vi "Project Data Initial for manual.vi"(10 "VISA resource name":refnum<visa-resource-name>="COM1", 11 "configuration file path":path=path "C:/Users/MyUser/Desktop/S2_Project.txt") -> (0 "error out":errorcluster, 1 "Step Content":string[][](table), 2 "Retry":i32, 3 "process cluster":cluster{string[], i32[]})   [LabVIEW 2019]
uses:
  <vilib>/Utility/config.llb/Read Key (String).vi
  Global/Process Global.vi
  <vilib>/Utility/config.llb/NI_LVConfig.lvlib
  Ctrl/StationCmdSelect.ctl
  FlowCtrl Class/LineScan/LineScan.lvclass
  Ctrl/MeasureDisplayTab.ctl
  LLB/Commonly VI/Main Glb.vi
  LLB/Commonly VI.lvlib
  Ctrl/Table Save.ctl
  Ctrl/Auto Inspection Station Name2.ctl
  Ctrl/Auto Inspection Data Name.ctl
  Ctrl/S2 Station IO.ctl
panel:
  out "ToolStringOut_P1_2":string
  out "P1 Receive":string[](array[string])
  out "ToolStringOut_P1":string
  out "Initial_ChkSum":string
  out "Array":string[](array[string])
  out "S1 ChkSum":string
  out "ToolStringOut_Init":string
  out "S1 ToolStringOut":string
  out "Initial receive 2":string
  out "result string 2":string
  out "Program receive 2":string
  out "S2 receive":string
  out "Blue Scan2 receive":string
  out "T2 buffer":string
  out "T2 μA":dbl format="%#_6f"
  out "T1 buffer":string
  out "T1 μA":dbl format="%#_6f"
  in  "error in (no error)":errorcluster
  out "Blue Scan receive":string
  out "S1 receive":string
  out "Program receive":string
  out "Initial receive":string
  out "Act Step":i32
  out "retry次數":string[](array[string])
  in  "stop":bool
  out "Boolean":bool=TRUE
  in  "Numeric 3":i32
  out "format receive":string
  out "CurrentCmd":string
  out "Numeric":dbl
  in  "Table Control":string[][](table)=[["PCBA BARCODE", ""], ["硬體(Tool初始化)", ""], ["company(Tool初始化)", ""], ["耗電流 uA(電流表)", "T"], ["電池負載電壓", "T"], ["晶片ID(Tool FORMAT)", "F"], ["雷雕ID(TOOl scan、藍芽接收器)", "S"], ["Format(Tool FORMAT)", "F"], ["Programe(Tool Programe)", "P"]]
  out "subarray":string[](array[string])
  out "array":string[](array[string])
  out "Process":string[](array[string])
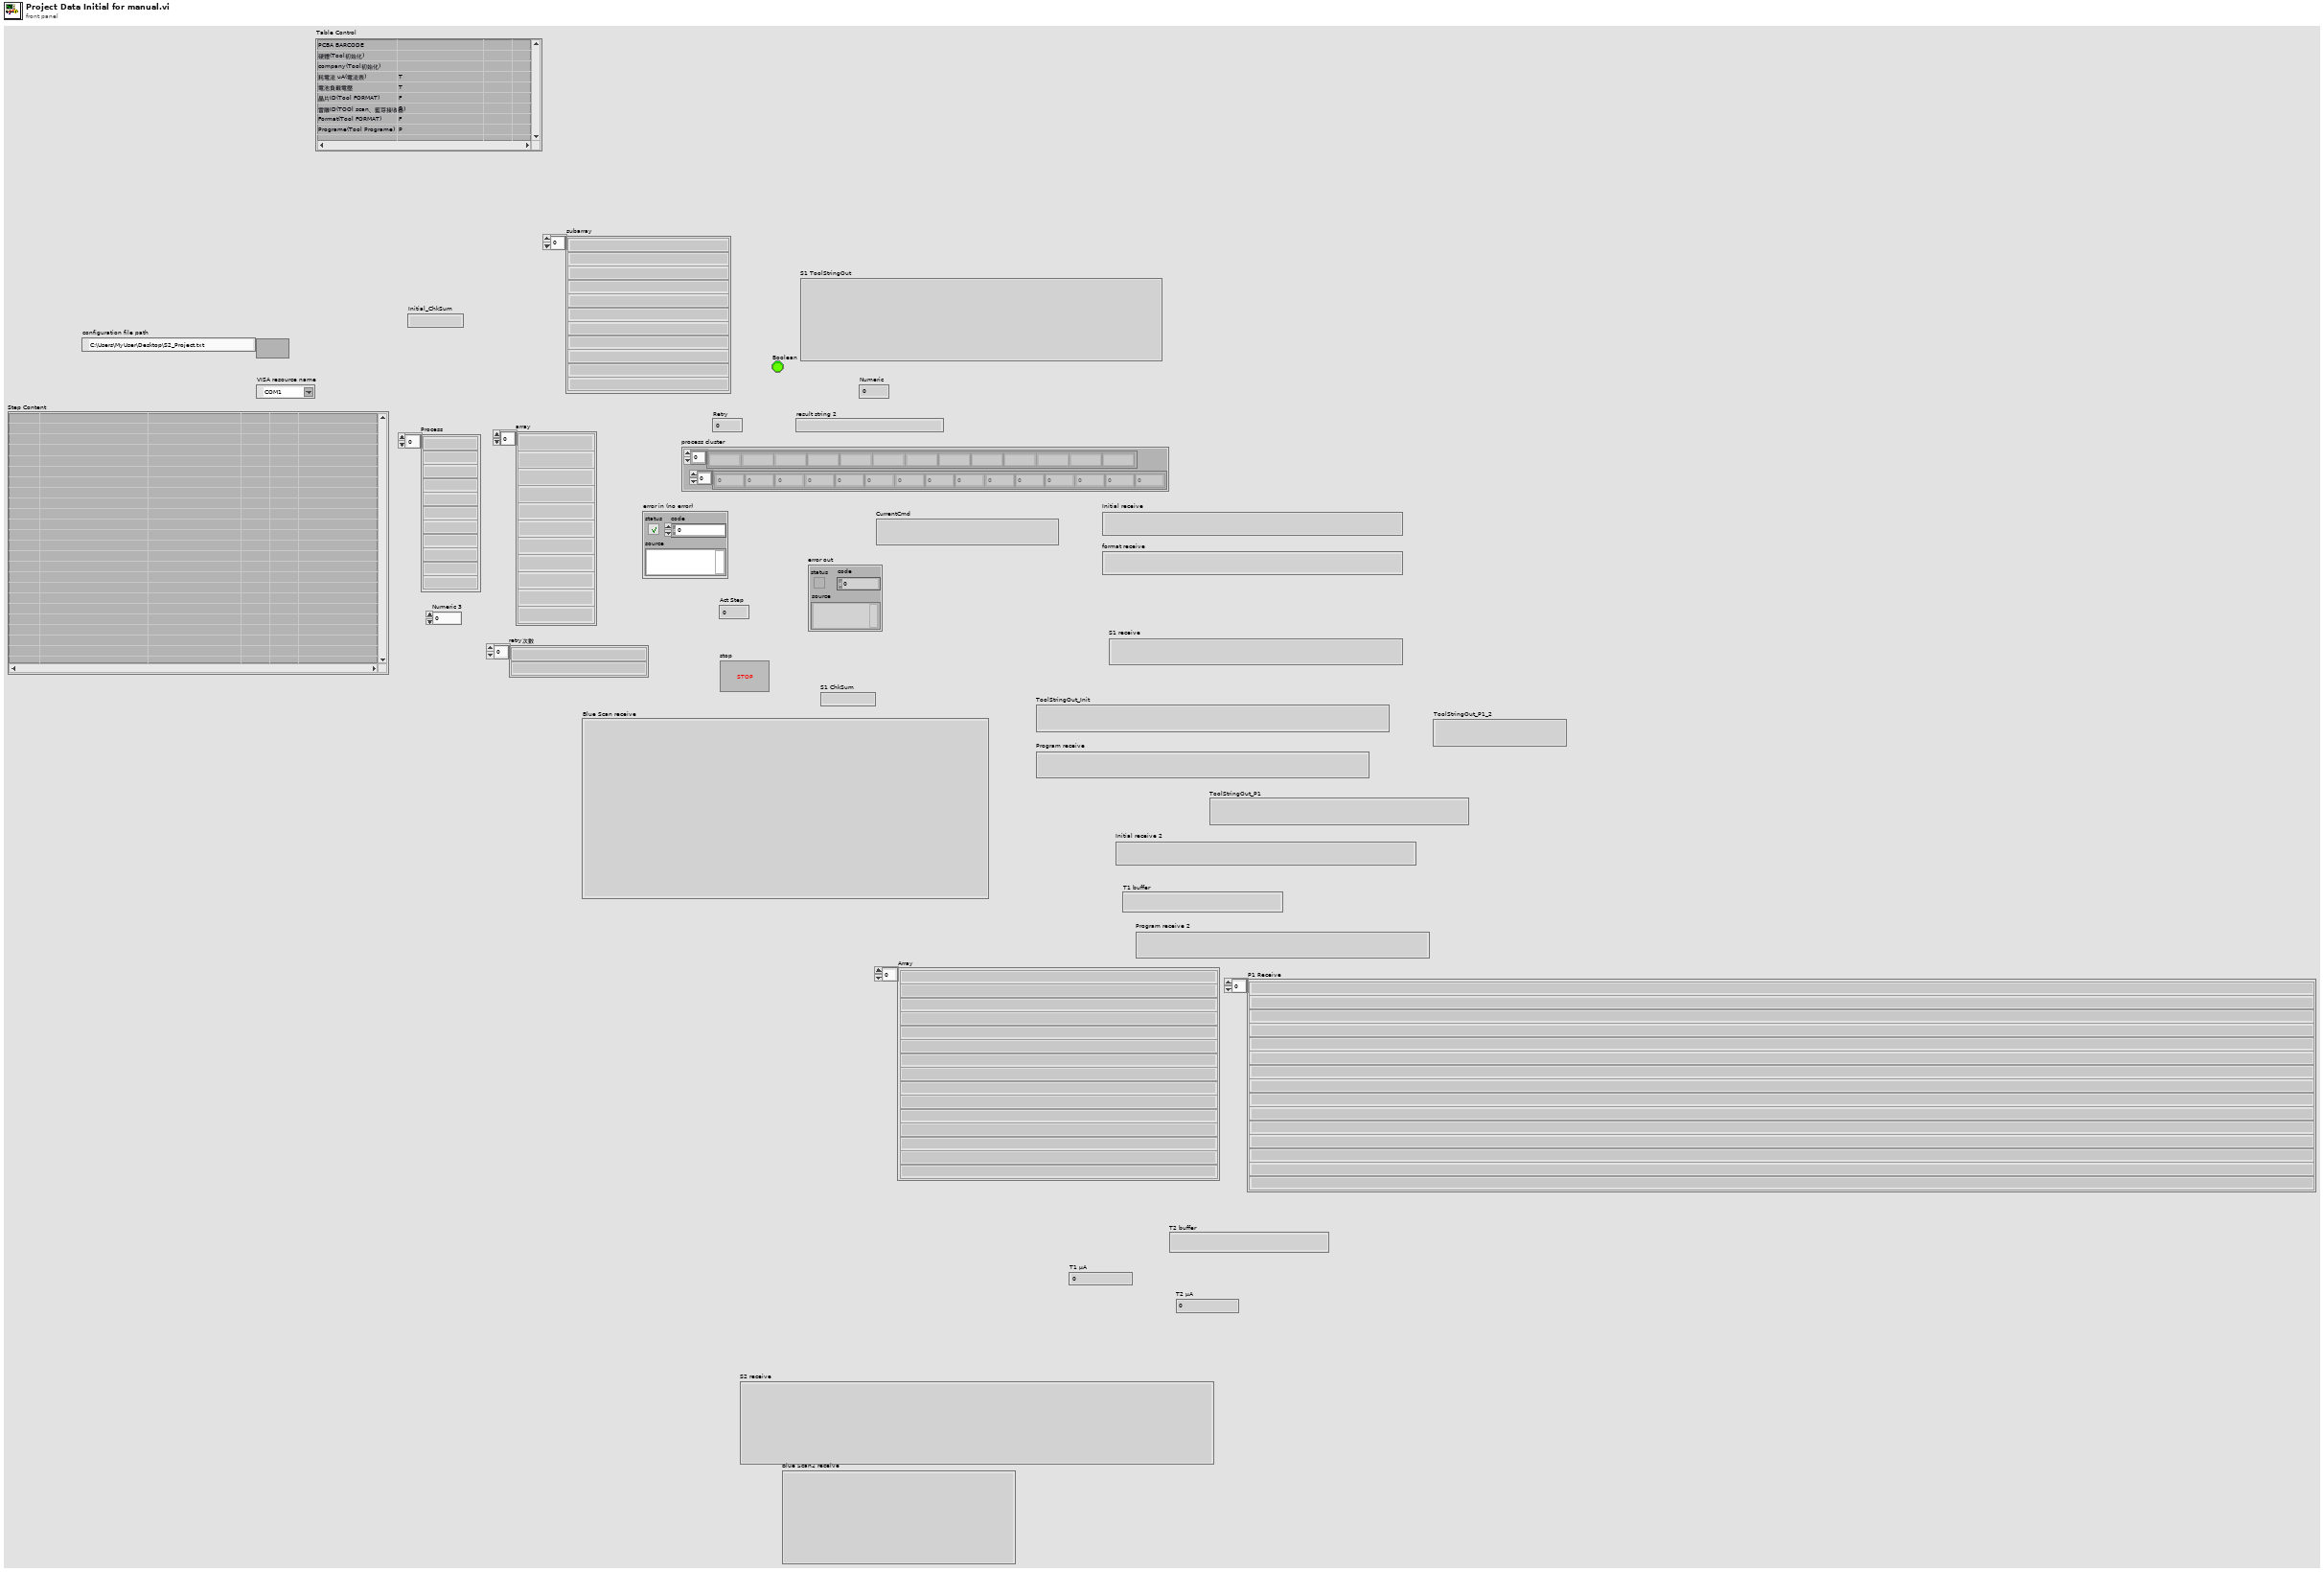
[diagram p1: front panel]
types:
  T1 = typedef "NI_LVConfig.lvlib/Config Data RefNum.ctl" = refnum<k1>
  T2 = typedef "StationCmdSelect.ctl" = enum16{"Action", "Command", "Return", "DTime", "Retry"}
  T3 = typedef "Auto Inspection Data Name.ctl" = enum16{"LocalRun", "ItemSN(TimeCode)", "CurrentAction", "Error", "Data", "OKNG", "電壓值", "電壓值判斷", "電流值", "電流值判斷", "Laser1 Data", "Laser2 Data", "Laser OKNG", "StationNO"}
  T4 = typedef "Auto Inspection Station Name2.ctl" = enum16{"S1Barcode", "S2Measure", "S3Measure", "S4Measure", "S5Measure", "S11_LaserCheck"}
  T5 = typedef "Table Save.ctl" = enum16{"initial", "Add", "Write", "Replace", "Delete", "REad", "RedTable", "Load"}
  T6 = typedef "MeasureDisplayTab.ctl" = enum16{"Tray Barcode", "PCBA BARCODE", "硬體(Tool初始化)", "company(Tool初始化)", "耗電流 uA(電流表)", "電池負載電壓", "晶片ID(Tool FORMAT)", "雷雕ID(TOOl scan、藍芽接收器)", "Format(Tool FORMAT)", "Programe(Tool Programe)", "MAC(藍芽接收器)", "ID(藍芽接收器)", "KPA(藍芽接收器)", "溫度(藍芽接收器)", "SENSOR電池電壓(藍芽接收器)", "RSSI(藍芽接收器)", "SensorType_315(FSK scan)", "FSKsnVol_315(FSK scan)", "FSKscanl_315(FSK scan)", "P_315(FSK scan)", "T_315(FSK scan)", "SensorType_433(ASK scan)", "ASKsnVol_433(ASK scan)", "ASKscan_433(ASK scan)", "P_433(ASK scan)", "T_433(ASK scan)", "測高Data"}
  T7 = typedef "S2 Station IO.ctl" = enum16{"S2站PC動作中_20", "電流量測完成產品OK_21", "電流量測完成產品NG_22", "S2站Format 執行_23", "S2 Format OK_24", "S2 Format NG_25", "S2站燒入執行_26", "S2站燒入OK_27", "S2站燒入NG_28", "S2站動作完成_29", "S3 PC動作中_30", "S3 Format 此站執行_31", "S3 Format OK_32", "S3 Format NG_33", "S3 燒入程式 此站執行_34", "S3 燒入程式 OK_35", "S3 燒入程式 NG_36", "S3 備用_37", "S3 備用_38", "S3 動作完成_39", "S4 PC動作中_40", "S4 量測完成 產品正常_41", "S4 量測完成 產品NG_42", "S4 Format 此站執行_43", "S4 Format OK_44", "S4 Format NG_45", "S4 燒入 此站不執行_46", "S4 燒入程式 OK_47", "S4 燒入程式 NG_48", "S4 藍芽Scan OK_49", "S4 藍芽Scan NG_50", "S4 動作完成_51", "給PLC要量電流訊號", "給PLC要量電壓訊號"}
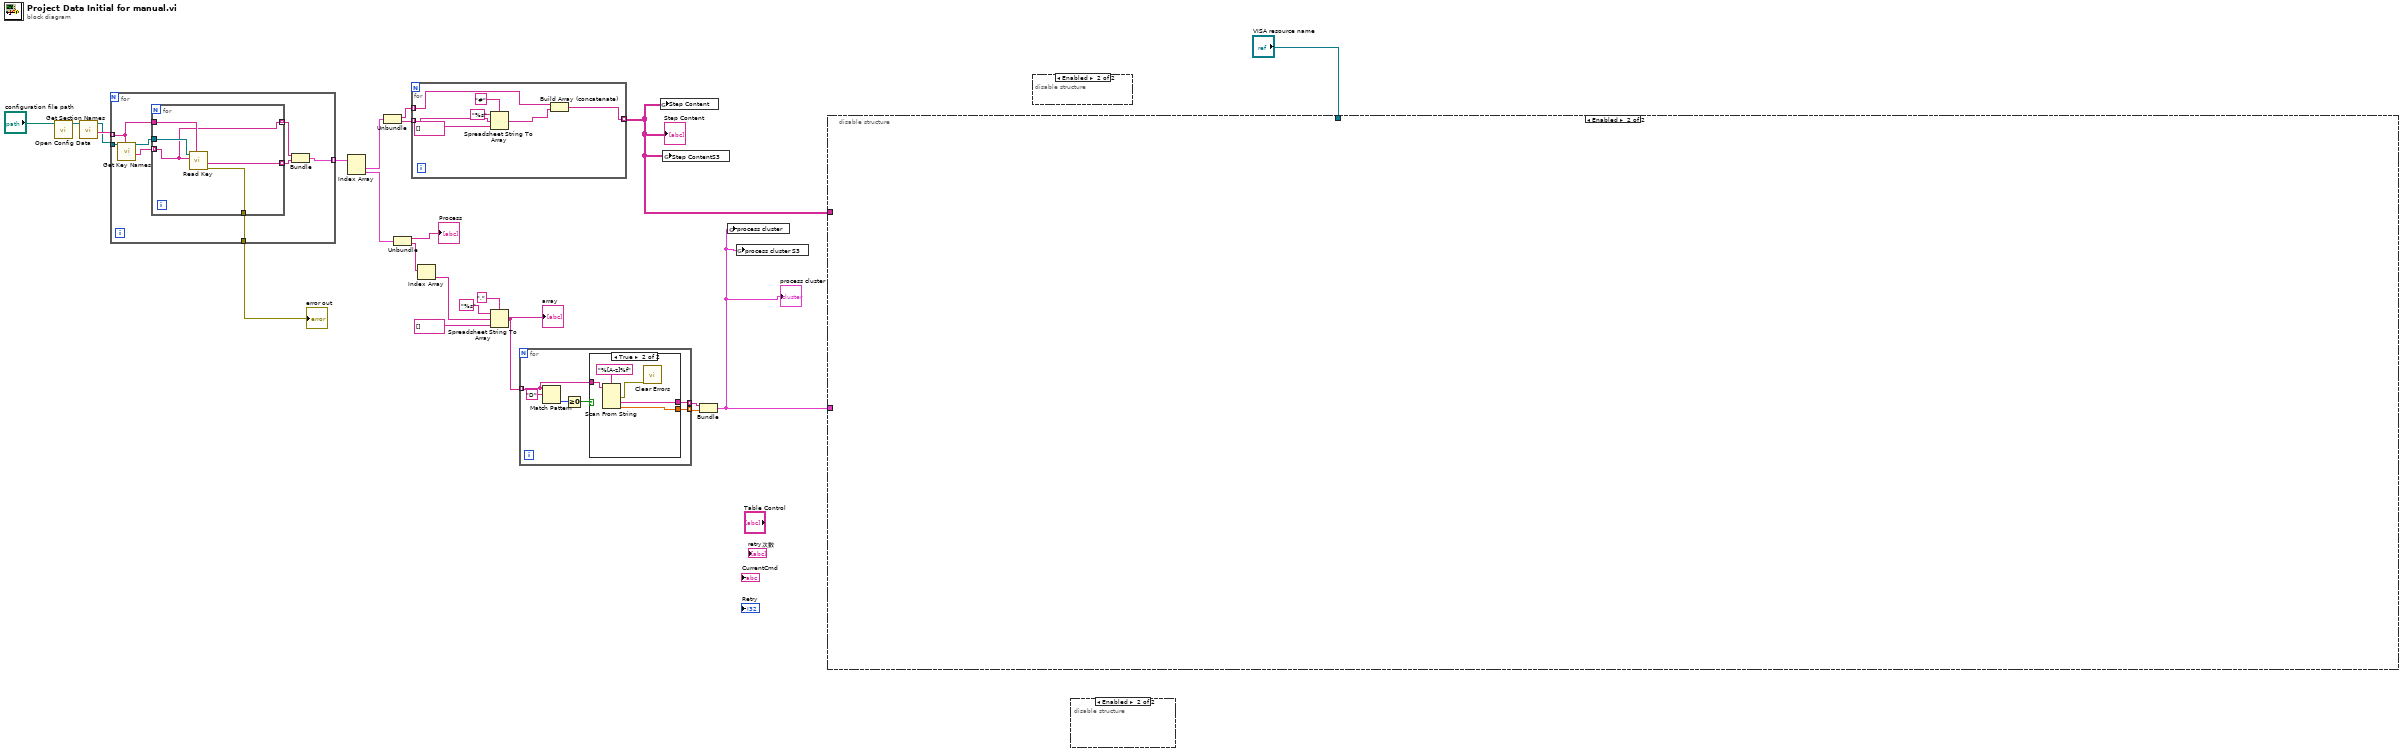
[diagram p0: block diagram]
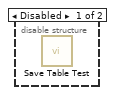
[diagram p2: hidden frame]
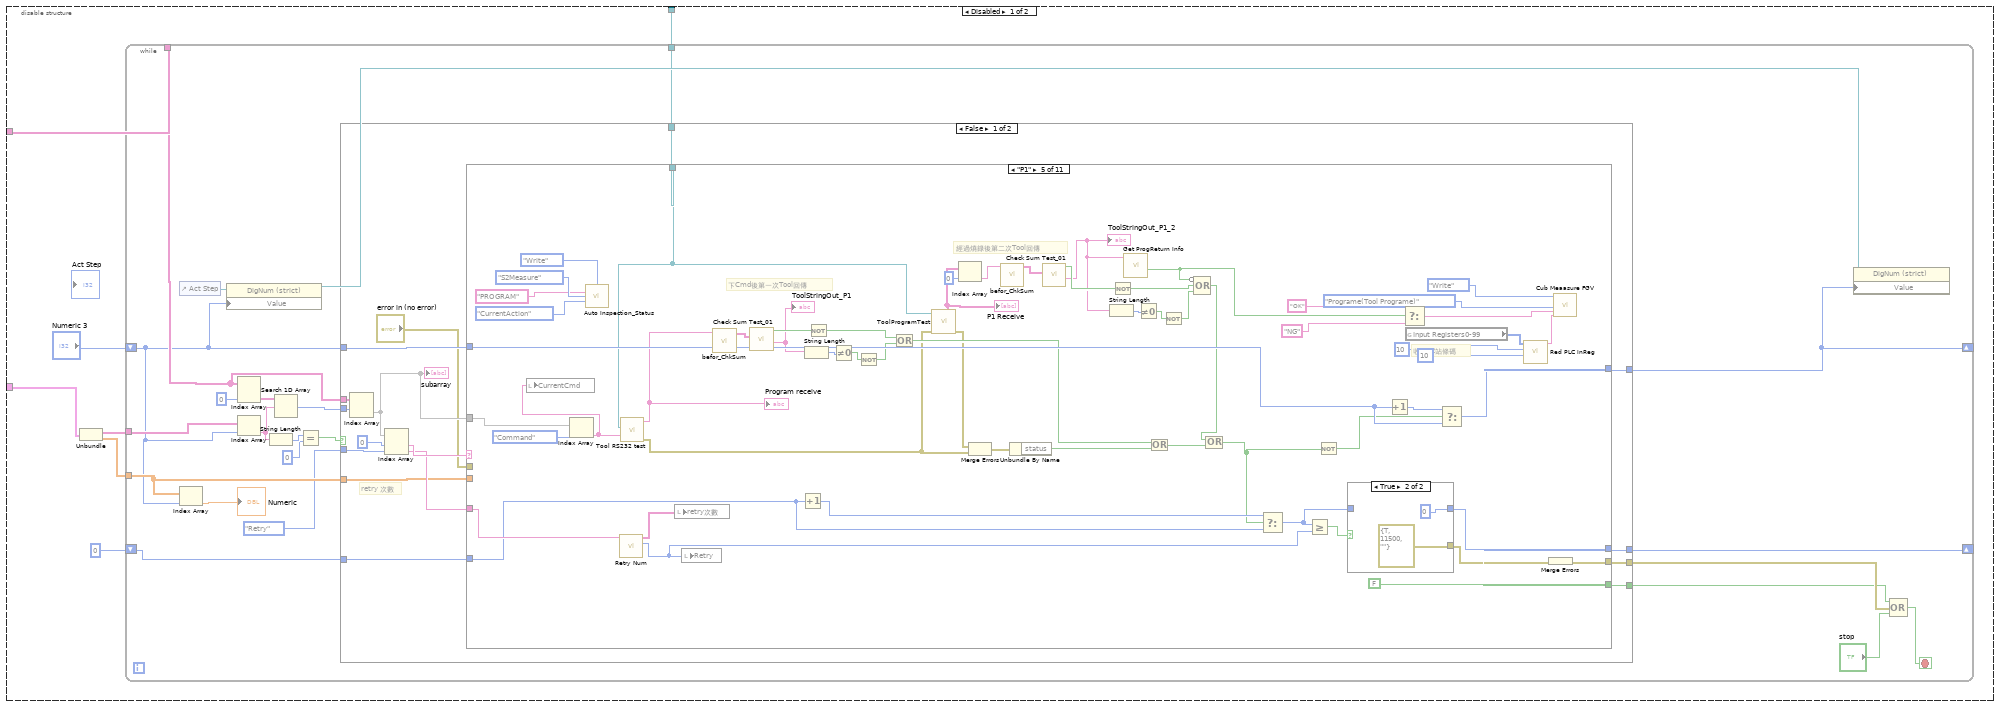
[diagram p3: hidden frame]
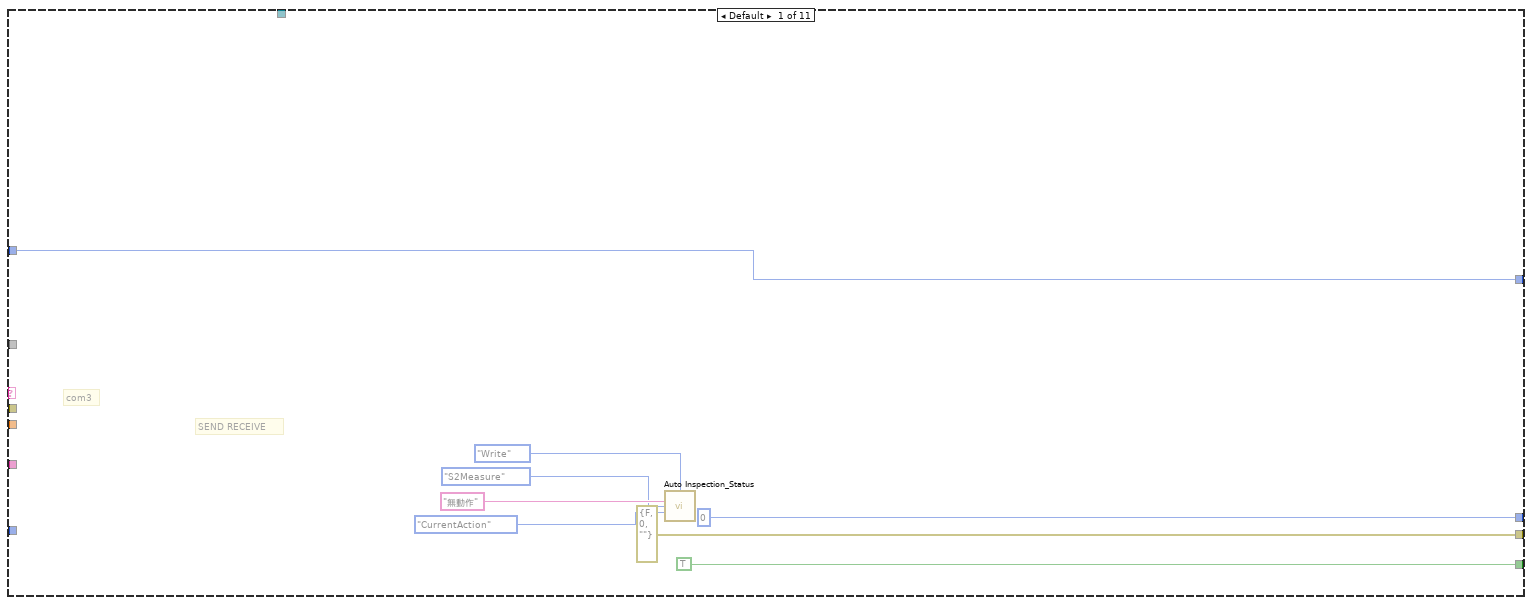
[diagram p4: hidden frame]
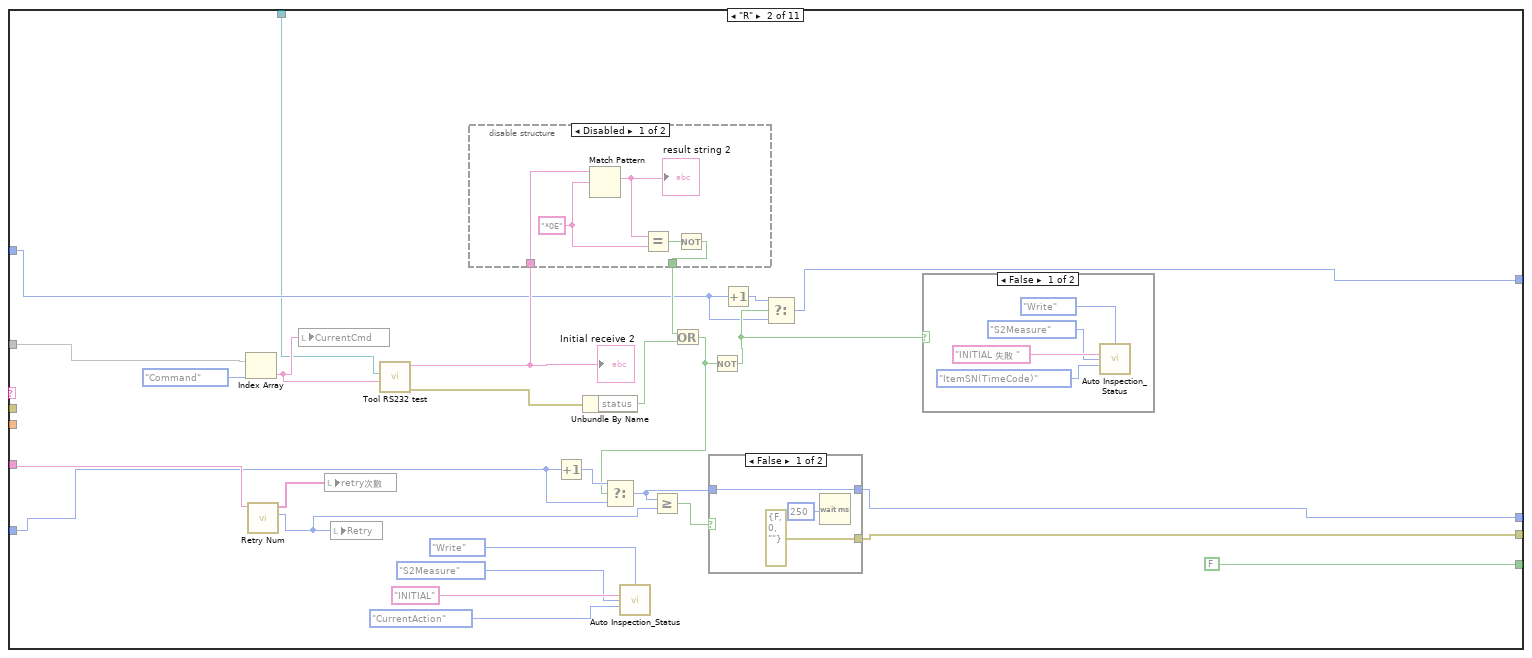
[diagram p5: hidden frame]
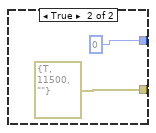
[diagram p8: hidden frame]
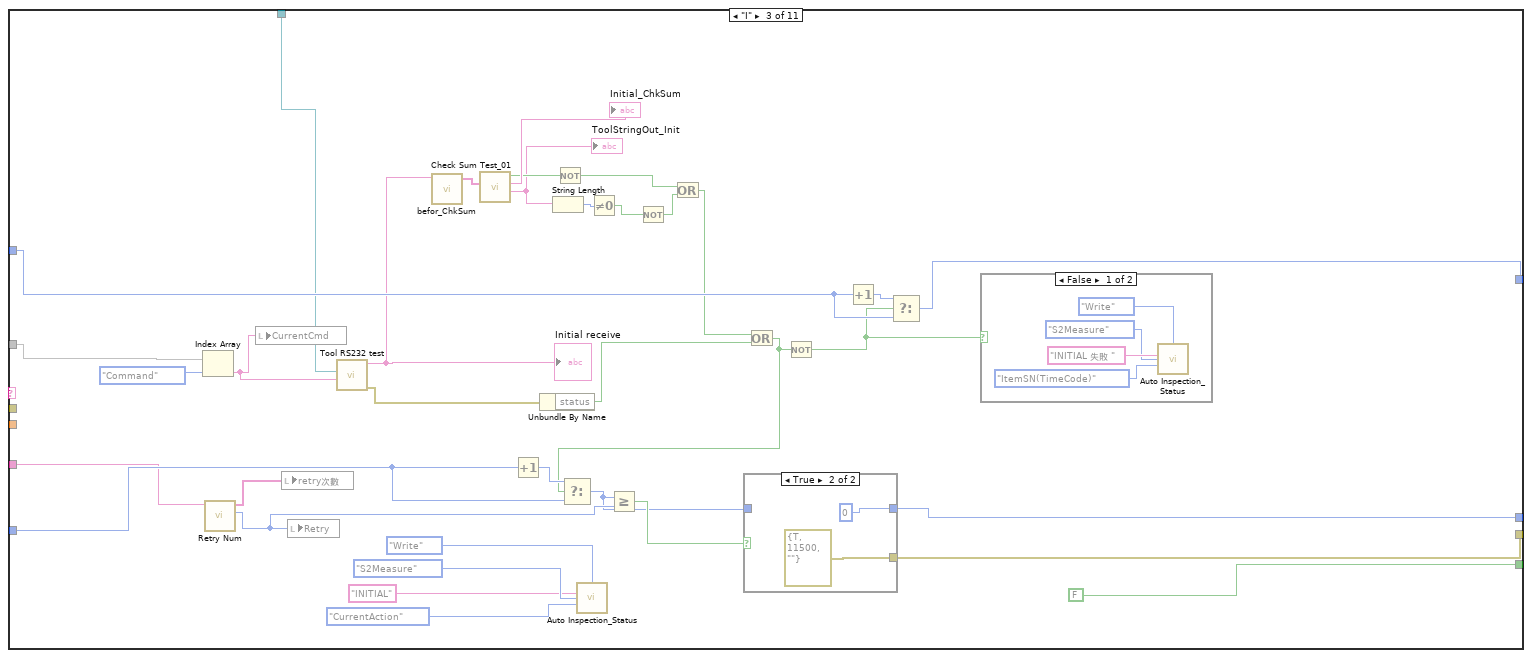
[diagram p9: hidden frame]
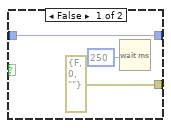
[diagram p11: hidden frame]
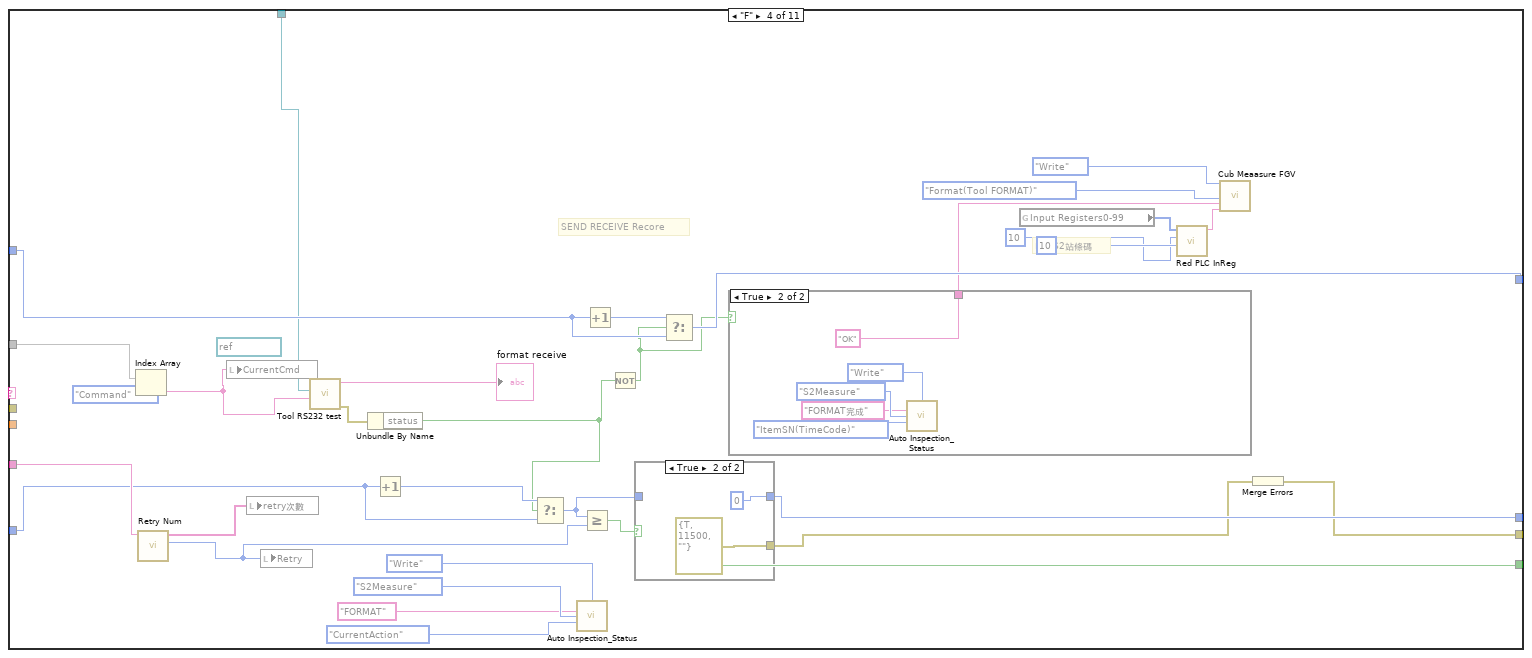
[diagram p12: hidden frame]
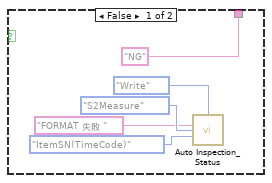
[diagram p13: hidden frame]
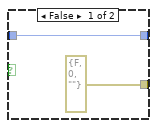
[diagram p14: hidden frame]
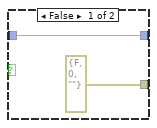
[diagram p15: hidden frame]
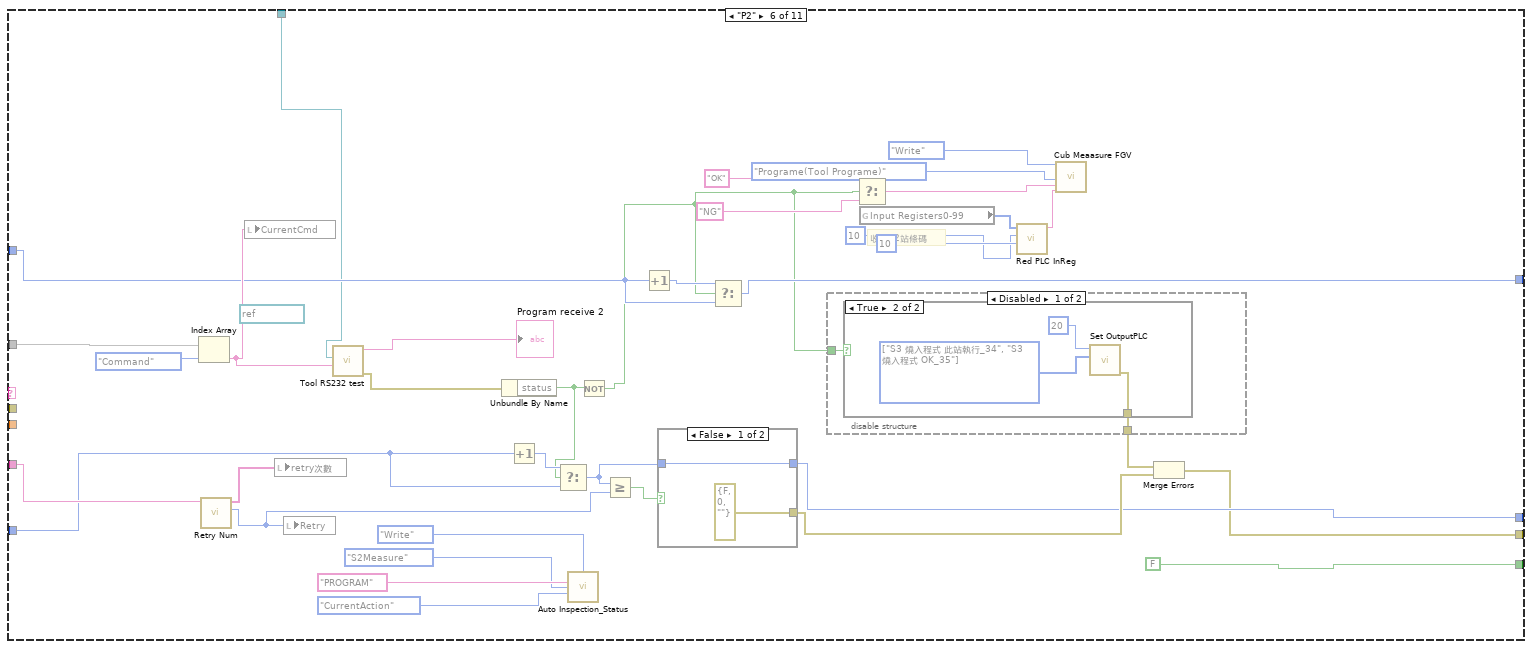
[diagram p16: hidden frame]
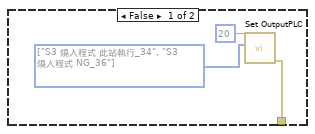
[diagram p17: hidden frame]
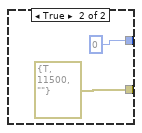
[diagram p19: hidden frame]
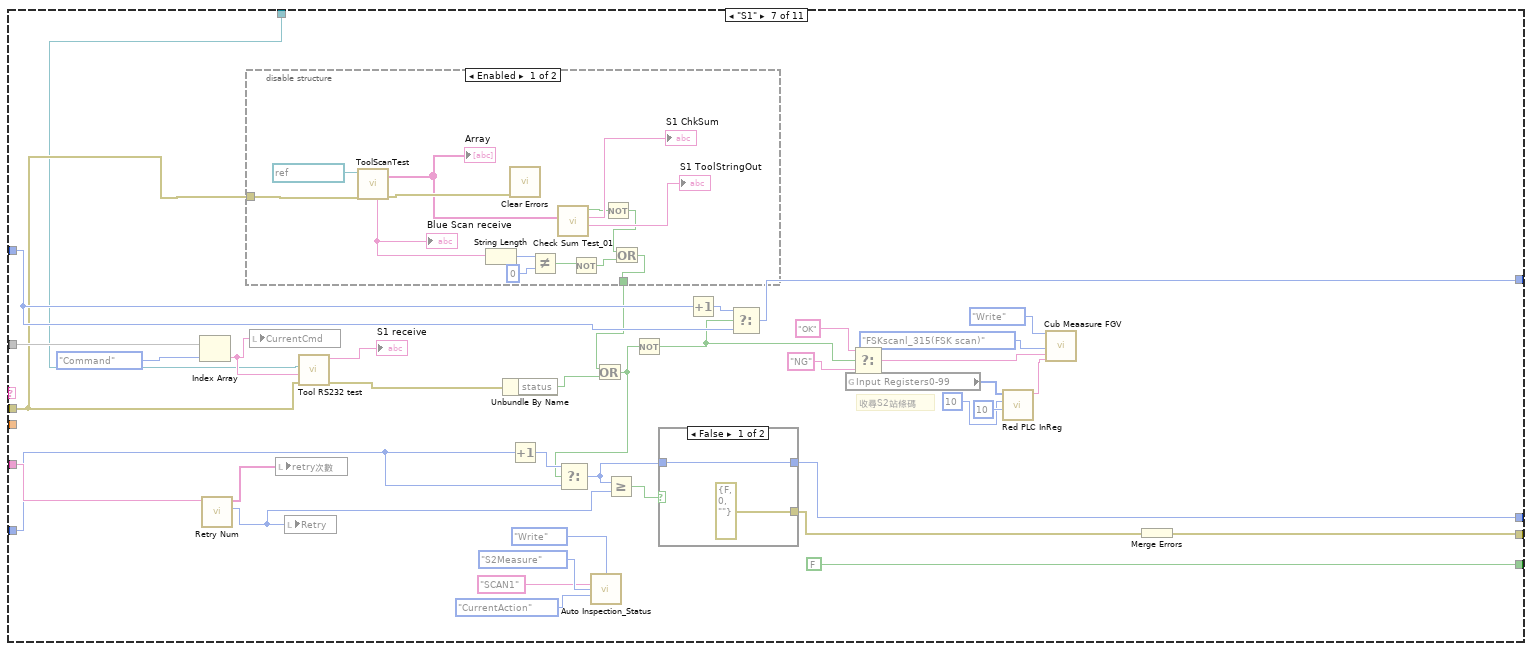
[diagram p20: hidden frame]
diagram:
  n1 = call <vilib>:"Open Config Data.vi"("configuration file path"="configuration file path") -> ("refnum"=w21:T1)  [unwired: 8 in, 2 out]
  n2 = call <vilib>:"Get Section Names.vi"("refnum"=w21) -> ("section names"=w20:string[], "refnum out"=w19:T1)  [unwired: 8 in, 1 out]
  n3 = for {
    tunnel: w19 -> [w30]
    tunnel: w20 -> [w25] mode=indexing
    tunnel: [w27] -> w17 mode=indexing
    tunnel: [w23] -> w3
    n4 = call <vilib>:"Get Key Names.vi"("section"=w25, "refnum"=w30) -> ("key names"=w29:string[], "refnum out"=w26:T1)  [unwired: 6 in, 2 out]
    n5 = for {
      tunnel: w29 -> [w32] mode=indexing
      tunnel: [w35] -> w28 mode=indexing
      tunnel: w26 -> [w34]
      tunnel: w25 -> [w33]
      tunnel: [w32] -> w24 mode=indexing
      tunnel: [w31] -> w23
      n6 = call-poly <vilib>:"Read Key.vi"("section"=w33, "key"=w32, "refnum"=w34) -> ("error out"=w31:errorcluster, "value"=w35:string)  [unwired: 5 in, 2 out]
    }
    n7 = Bundle(w24, w28) -> (w27:cluster{string[], string[]})  [unwired: 1 in]
  }
  "error out" <- w3
  n8 = Index Array(array=w17) -> (element #1=w13:cluster{string[], string[]}, element #2=w16:cluster{string[], string[]})  [unwired: 2 in]
  n9 = Unbundle(w13) -> (w14:string[], w15:string[])
  n10 = Unbundle(w16) -> (→"Process":string[], w9:string[])
  n11 = for {
    tunnel: w15 -> [w40] mode=indexing
    tunnel: [w36] -> w4 mode=indexing
    tunnel: w14 -> [w37] mode=indexing
    n12 = Spreadsheet String To Array(delimiter (Tab)="#", format string="%s", spreadsheet string=w40, array type (2D Dbl)=string[] []) -> (array=w38:string[])
    n13 = Build Array (concatenate)(w37, w38) -> (w36:string[])
  }
  "Step Content" <- w4
  n14 = Index Array(array=w9) -> (element=w8:string)  [unwired: 1 in]
  n15 = Spreadsheet String To Array(delimiter (Tab)=",", format string="%s", spreadsheet string=w8, array type (2D Dbl)=string[] []) -> (array=w7:string[])
  "array" <- w7
  n16 = for {
    tunnel: w7 -> [w43] mode=indexing
    tunnel: [w48] -> w6 mode=indexing
    tunnel: [w47] -> w5 mode=indexing
    n17 = Match Pattern(string=w43, regular expression="D") -> (offset past match=w45:i32)  [unwired: 1 in, 3 out]
    n18 = Greater Or Equal To 0?(x=w45) -> (x >= 0?=w44:bool)
    n19 = case shown="True" w44 {
      tunnel: [w50 w54] -> w48
      tunnel: [-1.0 w53] -> w47
      tunnel: w43 -> [w50 w51]
      frame False {
      }
      frame True {
        n20 = Scan From String(format string="%[A-z]%f", input string=w51) -> (error out=w52:errorcluster, output 1=w54:string, output 2=w53:dbl)  [unwired: 4 in, 2 out]
        n21 = call <vilib>:"Clear Errors.vi"("error in (no error)"=w52) -> ()  [unwired: 5 in, 2 out]
      }
    }
  }
  n22 = global write "Process Global.vi" "Step Content"(w4) -> ()
  n23 = global write "Process Global.vi" "Step ContentS3"(w4) -> ()
  n24 = Bundle(w6, w5) -> (w1:cluster{string[], dbl[]})  [unwired: 1 in]
  "process cluster" <- w1
  n25 = global write "Process Global.vi" "process cluster"(w1) -> ()
  n26 = global write "Process Global.vi" "process cluster S3"(w1) -> ()
  n27 = disable-structure shown="Enabled" {
    disable-tunnel: w4 -> [w60 _]
    disable-tunnel: w1 -> [w59 _]
    disable-tunnel: "VISA resource name" -> [w56 _]
    frame Disabled {
      n28 = Unbundle(w59) -> (w62:string[], w61:dbl[])
      n29 = while {
        tunnel: w62 -> [w85]
        tunnel: w61 -> [w84]
        tunnel: w60 -> [w83]
        shift-right: [w66] -> _
        shift-left: 0 -> [w70]
        shift-right: [w67] -> _
        shift-left: "Numeric 3" -> [w64]
        tunnel: w56 -> [w63]
        stop <- w71 stop-if-true
        n30 = control-ref of="Act Step"() -> (w69:refnum<vi>)
        n31 = Index Array(array=w84, index=w64) -> (element=→"Numeric":dbl)
        n32 = property class="DigNum (strict)"(reference=w69, "Value"=w64) -> (reference out=w68:refnum<vi>)  [unwired: 1 in, 1 out]
        n33 = Index Array(array=w83, index (col)=0 ("disabled index (col)")) -> (element=w81:string[])  [unwired: 1 in]
        n34 = Index Array(array=w85, index=w64) -> (element=w78:string)
        n35 = String Length(string=w78) -> (length=w77:i32)
        n36 = Search 1D Array(1D array=w81, element=w78) -> (index of element=w80:i32)  [unwired: 1 in]
        n37 = Equal?(x=w77, y=0) -> (x = y?=w75:bool)
        n38 = case shown="False" w75 {
          tunnel: w83 -> [w101 _]
          tunnel: w80 -> [w100 _]
          tunnel: w84 -> [w96 _]
          tunnel: w70 -> [w94 _]
          tunnel: StationCmdSelect."Retry" -> [w93 _]
          tunnel: [w92 _] -> w72
          tunnel: w64 -> [w91 _]
          tunnel: [w90 _] -> w67
          tunnel: [w89 _] -> w66
          tunnel: [w88 w574] -> w65
          tunnel: w63 -> [w86 _]
          frame False {
            # "retry 次數"
            n39 = Index Array(array=w101, index (row)=w100) -> (element=w95:string[])  [unwired: 1 in]
            "subarray" <- w95
            n40 = Index Array(array=w95, index #1=0 ("index"), index #2=w93) -> (element #1=w98:string, element #2=w97:string)
            n41 = case shown="\"P1\"" w98 {
              tunnel: w96 -> [_ _ _ _ _ _ _ _ w476 _ _]
              tunnel: w97 -> [_ w117 w173 w224 w290 w315 w379 w435 _ w498 w545]
              tunnel: w95 -> [_ w118 w175 w227 w289 w313 w376 w436 _ _ _]
              tunnel: w94 -> [_ w116 w174 w221 w287 w314 w374 w434 w473 w499 w546]
              tunnel: [errorcluster {"status"=FALSE, "code"=0, "source"=""} ("error constant") w113 w178 w198 w270 w309 w358 w413 _ w480 w529] -> w92
              tunnel: w91 -> [w109 w119 w176 w217 w286 w312 w378 w438 w471 w497 w547]
              tunnel: [w109 w112 w172 w216 w292 w311 w377 w431 w470 w496 w548] -> w90
              tunnel: [0 w115 w177 w214 w291 w310 w380 w433 _ w495 w550] -> w89
              tunnel: [TRUE FALSE FALSE FALSE FALSE FALSE FALSE FALSE FALSE FALSE FALSE] -> w88
              tunnel: "error in (no error)" -> [_ _ _ _ _ _ w355 w437 _ _ _]
              tunnel: w86 -> [_ w111 w161 w195 w269 w305 w354 w410 _ _ _]
              frame Default {
                # "SEND RECEIVE"
                # "com3"
                n42 = call "Auto Inspection_Status.vi"("Action"=enum16{"Initial", "Write", "Read"}."Write", "DataIn"="無動作", "Station"=Auto_Inspection_Station_Name2."S2Measure", "Data"=Auto_Inspection_Data_Name."CurrentAction") -> ()  [unwired: 9 in, 3 out]
              }
              frame "R" {
                n43 = Index Array(array=w118, index=StationCmdSelect."Command") -> (element=w129:string)
                n44 = call "Retry Num.vi"("String"=w117) -> ("Numeric"=w134:i32, "retry次數"=w130:string[])  [unwired: 9 in]
                n45 = local write "CurrentCmd"(w129) -> ()
                n46 = local write "retry次數"(w130) -> ()
                n47 = local write "Retry"(w134) -> ()
                n48 = call "Tool RS232 test.vi"("Cmd In"=w129, "VISA resource name"=w111) -> ("error out"=w135:errorcluster, "receive string"=w126:string)  [unwired: 8 in]
                "Initial receive 2" <- w126
                n49 = disable-structure shown="Disabled" {
                  disable-tunnel: [w140 _] -> w128
                  disable-tunnel: w126 -> [w139 _]
                  frame Disabled {
                    w137 = "*0E" ("search string")
                    n50 = Match Pattern(string=w139, regular expression=w137) -> (match substring=w138:string)  [unwired: 1 in, 3 out]
                    "result string 2" <- w138
                    n51 = Equal?(x=w138, y=w137) -> (x = y?=w141:bool)
                    n52 = Not(x=w141) -> (.not. x?=w140:bool)
                  }
                  frame Enabled {
                  }
                }
                n53 = Increment(x=w116) -> (x+1=w136:i32)
                n54 = Unbundle By Name(w135) -> ("status"=w127:bool)
                n55 = call "Auto Inspection_Status.vi"("Action"=enum16{"Initial", "Write", "Read"}."Write", "DataIn"="INITIAL", "Station"=Auto_Inspection_Station_Name2."S2Measure", "Data"=Auto_Inspection_Data_Name."CurrentAction") -> ()  [unwired: 9 in, 3 out]
                n56 = Or(x=w128, y=w127) -> (x .or. y?=w110:bool)
                n57 = Select(t=w136, s=w110, f=w116) -> (s? t:f=w131:i32)
                n58 = Greater Or Equal?(x=w131, y=w134) -> (x >= y?=w133:bool)
                n59 = case shown="False" w133 {
                  tunnel: [errorcluster {"status"=FALSE, "code"=0, "source"=""} ("error constant") errorcluster {"status"=TRUE, "code"=11500, "source"=""} ("error constant")] -> w113
                  tunnel: w131 -> [w147 _]
                  tunnel: [w147 0] -> w115
                  frame False {
                    n60 = Wait (ms)(milliseconds to wait=250) -> ()  [unwired: 1 out]
                  }
                  frame True {
                  }
                }
                n61 = Not(x=w110) -> (.not. x?=w125:bool)
                n62 = Increment(x=w119) -> (x+1=w132:i32)
                n63 = Select(t=w132, s=w125, f=w119) -> (s? t:f=w112:i32)
                n64 = case shown="False" w125 {
                  frame False {
                    n65 = call "Auto Inspection_Status.vi"("Action"=enum16{"Initial", "Write", "Read"}."Write", "DataIn"="INITIAL 失敗 ", "Station"=Auto_Inspection_Station_Name2."S2Measure", "Data"=Auto_Inspection_Data_Name."ItemSN(TimeCode)") -> ()  [unwired: 9 in, 3 out]
                  }
                  frame True {
                  }
                }
              }
              frame "I" {
                n66 = Index Array(array=w175, index=StationCmdSelect."Command") -> (element=w170:string)
                n67 = call "Retry Num.vi"("String"=w173) -> ("Numeric"=w183:i32, "retry次數"=w171:string[])  [unwired: 9 in]
                n68 = local write "CurrentCmd"(w170) -> ()
                n69 = local write "retry次數"(w171) -> ()
                n70 = local write "Retry"(w183) -> ()
                n71 = call "Tool RS232 test.vi"("Cmd In"=w170, "VISA resource name"=w161) -> ("error out"=w184:errorcluster, "receive string"=w158:string)  [unwired: 8 in]
                "Initial receive" <- w158
                n72 = call "befor_ChkSum.vi"("ToolString Input"=w158) -> ("Array"=w157:string[])  [unwired: 9 in, 1 out]
                n73 = call "Check Sum Test_01.vi"("Array"=w157) -> ("ToolStringOut_01"=w154:string, "ChkSum"=→"Initial_ChkSum":string, "x = y?"=w156:bool)  [unwired: 8 in]
                "ToolStringOut_Init" <- w154
                n74 = Increment(x=w174) -> (x+1=w185:i32)
                n75 = Unbundle By Name(w184) -> ("status"=w164:bool)
                n76 = String Length(string=w154) -> (length=w152:i32)
                n77 = Not(x=w156) -> (.not. x?=w155:bool)
                n78 = call "Auto Inspection_Status.vi"("Action"=enum16{"Initial", "Write", "Read"}."Write", "DataIn"="INITIAL", "Station"=Auto_Inspection_Station_Name2."S2Measure", "Data"=Auto_Inspection_Data_Name."CurrentAction") -> ()  [unwired: 9 in, 3 out]
                n79 = Not Equal To 0?(x=w152) -> (x != 0?=w151:bool)
                n80 = Not(x=w151) -> (.not. x?=w153:bool)
                n81 = Or(x=w155, y=w153) -> (x .or. y?=w160:bool)
                n82 = Or(x=w160, y=w164) -> (x .or. y?=w162:bool)
                n83 = Select(t=w185, s=w162, f=w174) -> (s? t:f=w180:i32)
                n84 = Greater Or Equal?(x=w180, y=w183) -> (x >= y?=w182:bool)
                n85 = case shown="True" w182 {
                  tunnel: [errorcluster {"status"=FALSE, "code"=0, "source"=""} ("error constant") errorcluster {"status"=TRUE, "code"=11500, "source"=""} ("error constant")] -> w178
                  tunnel: w180 -> [w191 _]
                  tunnel: [w191 0] -> w177
                  frame False {
                    n86 = Wait (ms)(milliseconds to wait=250) -> ()  [unwired: 1 out]
                  }
                  frame True {
                  }
                }
                n87 = Not(x=w162) -> (.not. x?=w163:bool)
                n88 = Increment(x=w176) -> (x+1=w181:i32)
                n89 = Select(t=w181, s=w163, f=w176) -> (s? t:f=w172:i32)
                n90 = case shown="False" w163 {
                  frame False {
                    n91 = call "Auto Inspection_Status.vi"("Action"=enum16{"Initial", "Write", "Read"}."Write", "DataIn"="INITIAL 失敗 ", "Station"=Auto_Inspection_Station_Name2."S2Measure", "Data"=Auto_Inspection_Data_Name."ItemSN(TimeCode)") -> ()  [unwired: 9 in, 3 out]
                  }
                  frame True {
                  }
                }
              }
              frame "F" {
                (unwired) refnum<visa-resource-name> "COM1" ("VISA resource name")
                # "收尋S2站條碼"
                # "SEND RECEIVE Recore"
                n92 = Index Array(array=w227, index=StationCmdSelect."Command") -> (element=w213:string)
                n93 = call "Retry Num.vi"("String"=w224) -> ("Numeric"=w220:i32, "retry次數"=w212:string[])  [unwired: 9 in]
                n94 = local write "CurrentCmd"(w213) -> ()
                n95 = local write "retry次數"(w212) -> ()
                n96 = local write "Retry"(w220) -> ()
                n97 = call "Tool RS232 test.vi"("Cmd In"=w213, "VISA resource name"=w195) -> ("error out"=w222:errorcluster, "receive string"=→"format receive":string)  [unwired: 8 in]
                n98 = Unbundle By Name(w222) -> ("status"=w196:bool)
                n99 = Increment(x=w221) -> (x+1=w223:i32)
                n100 = Select(t=w223, s=w196, f=w221) -> (s? t:f=w215:i32)
                n101 = call "Auto Inspection_Status.vi"("Action"=enum16{"Initial", "Write", "Read"}."Write", "DataIn"="FORMAT", "Station"=Auto_Inspection_Station_Name2."S2Measure", "Data"=Auto_Inspection_Data_Name."CurrentAction") -> ()  [unwired: 9 in, 3 out]
                n102 = Greater Or Equal?(x=w215, y=w220) -> (x >= y?=w219:bool)
                n103 = Increment(x=w217) -> (x+1=w218:i32)
                n104 = Not(x=w196) -> (.not. x?=w197:bool)
                n105 = case shown="True" w219 {
                  tunnel: [errorcluster {"status"=FALSE, "code"=0, "source"=""} ("error constant") errorcluster {"status"=TRUE, "code"=11500, "source"=""} ("error constant")] -> w199
                  tunnel: w215 -> [w238 _]
                  tunnel: [w238 0] -> w214
                  frame False {
                  }
                  frame True {
                  }
                }
                n106 = Select(t=w218, s=w197, f=w217) -> (s? t:f=w216:i32)
                n107 = case shown="True" w197 {
                  tunnel: ["NG" "OK"] -> w204
                  frame False {
                    n108 = call "Auto Inspection_Status.vi"("Action"=enum16{"Initial", "Write", "Read"}."Write", "DataIn"="FORMAT 失敗 ", "Station"=Auto_Inspection_Station_Name2."S2Measure", "Data"=Auto_Inspection_Data_Name."ItemSN(TimeCode)") -> ()  [unwired: 9 in, 3 out]
                  }
                  frame True {
                    n109 = call "Auto Inspection_Status.vi"("Action"=enum16{"Initial", "Write", "Read"}."Write", "DataIn"="FORMAT完成", "Station"=Auto_Inspection_Station_Name2."S2Measure", "Data"=Auto_Inspection_Data_Name."ItemSN(TimeCode)") -> ()  [unwired: 9 in, 3 out]
                  }
                }
                n110 = global read "Main Glb.vi" "Input Registers0-99"() -> (w203:u16[])
                n111 = call "Red PLC InReg.vi"("length"=10, "index"=10, "Input Registers Arr"=w203) -> ("Rad In Reg"=w200:string)  [unwired: 7 in, 1 out]
                n112 = call "Cub Meaasure FGV.vi"("Action"=Table_Save."Write" ("Enum"), "Save Index"=MeasureDisplayTab."Format(Tool FORMAT)", "DataIn"=w204, "SN"=w200) -> ()  [unwired: 8 in, 8 out]
                n113 = Merge Errors(w199) -> (w198:errorcluster)
              }
              frame "P1" {
                # "經過燒錄後第二次Tool回傳"
                # "下Cmd後第一次Tool回傳"
                # "收尋S2站條碼"
                n114 = Index Array(array=w289, index=StationCmdSelect."Command") -> (element=w300:string)
                n115 = local write "CurrentCmd"(w300) -> ()
                n116 = call "Auto Inspection_Status.vi"("Action"=enum16{"Initial", "Write", "Read"}."Write", "DataIn"="PROGRAM", "Station"=Auto_Inspection_Station_Name2."S2Measure", "Data"=Auto_Inspection_Data_Name."CurrentAction") -> ()  [unwired: 9 in, 3 out]
                n117 = call "Retry Num.vi"("String"=w290) -> ("Numeric"=w297:i32, "retry次數"=w299:string[])  [unwired: 9 in]
                n118 = call "Tool RS232 test.vi"("Cmd In"=w300, "VISA resource name"=w269) -> ("error out"=w259:errorcluster, "receive string"=w271:string)  [unwired: 8 in]
                "Program receive" <- w271
                n119 = local write "retry次數"(w299) -> ()
                n120 = local write "Retry"(w297) -> ()
                n121 = call "befor_ChkSum.vi"("ToolString Input"=w271) -> ("Array"=w280:string[])  [unwired: 9 in, 1 out]
                n122 = call "Check Sum Test_01.vi"("Array"=w280) -> ("ToolStringOut_01"=w277:string, "x = y?"=w279:bool)  [unwired: 8 in, 1 out]
                "ToolStringOut_P1" <- w277
                n123 = Increment(x=w287) -> (x+1=w298:i32)
                n124 = String Length(string=w277) -> (length=w275:i32)
                n125 = Not(x=w279) -> (.not. x?=w278:bool)
                n126 = Not Equal To 0?(x=w275) -> (x != 0?=w274:bool)
                n127 = Not(x=w274) -> (.not. x?=w276:bool)
                n128 = Or(x=w278, y=w276) -> (x .or. y?=w273:bool)
                n129 = call "ToolProgramTest.vi"("error in (no error)"=w259, "VISA resource name"=w269) -> ("error out"=w258:errorcluster, "Array"=w255:string[])  [unwired: 4 in, 4 out]
                "P1 Receive" <- w255
                n130 = Index Array(array=w255, index=0) -> (element=w253:string)
                n131 = Merge Errors(w258, w259) -> (w257:errorcluster)
                n132 = call "befor_ChkSum.vi"("ToolString Input"=w253) -> ("Array"=w252:string[])  [unwired: 9 in, 1 out]
                n133 = Unbundle By Name(w257) -> ("status"=w272:bool)
                n134 = call "Check Sum Test_01.vi"("Array"=w252) -> ("ToolStringOut_01"=w248:string, "x = y?"=w249:bool)  [unwired: 8 in, 1 out]
                "ToolStringOut_P1_2" <- w248
                n135 = String Length(string=w248) -> (length=w250:i32)
                n136 = Not(x=w249) -> (.not. x?=w245:bool)
                n137 = call "Get ProgReturn Info.vi"("String"=w248) -> ("Chk OK or Fail"=w242:bool)  [unwired: 8 in, 2 out]
                n138 = Not Equal To 0?(x=w250) -> (x != 0?=w251:bool)
                n139 = Or(x=w273, y=w272) -> (x .or. y?=w247:bool)
                n140 = Not(x=w251) -> (.not. x?=w244:bool)
                n141 = Compound Arithmetic op=OR(invert w242, w245, w244) -> (w243:bool)
                n142 = Compound Arithmetic op=OR(w243, w247) -> (w246:bool)
                n143 = Select(t=w298, s=w246, f=w287) -> (s? t:f=w294:i32)
                n144 = Greater Or Equal?(x=w294, y=w297) -> (x >= y?=w296:bool)
                n145 = Not(x=w246) -> (.not. x?=w256:bool)
                n146 = case shown="True" w296 {
                  tunnel: [errorcluster {"status"=FALSE, "code"=0, "source"=""} ("error constant") errorcluster {"status"=TRUE, "code"=11500, "source"=""} ("error constant")] -> w281
                  tunnel: w294 -> [w301 _]
                  tunnel: [w301 0] -> w291
                  frame False {
                  }
                  frame True {
                  }
                }
                n147 = Increment(x=w286) -> (x+1=w295:i32)
                n148 = Select(t="OK" ("DataIn"), s=w242, f="NG" ("DataIn")) -> (s? t:f=w266:string)
                n149 = global read "Main Glb.vi" "Input Registers0-99"() -> (w268:u16[])
                n150 = Select(t=w295, s=w256, f=w286) -> (s? t:f=w292:i32)
                n151 = call "Red PLC InReg.vi"("length"=10, "index"=10, "Input Registers Arr"=w268) -> ("Rad In Reg"=w267:string)  [unwired: 7 in, 1 out]
                n152 = Merge Errors(w281) -> (w270:errorcluster)
                n153 = call "Cub Meaasure FGV.vi"("Action"=Table_Save."Write" ("Enum"), "Save Index"=MeasureDisplayTab."Programe(Tool Programe)", "DataIn"=w266, "SN"=w267) -> ()  [unwired: 8 in, 8 out]
              }
              frame "P2" {
                (unwired) refnum<visa-resource-name> "COM1" ("VISA resource name")
                # "收尋S2站條碼"
                n154 = Index Array(array=w313, index=StationCmdSelect."Command") -> (element=w340:string)
                n155 = call "Retry Num.vi"("String"=w315) -> ("Numeric"=w335:i32, "retry次數"=w339:string[])  [unwired: 9 in]
                n156 = local write "CurrentCmd"(w340) -> ()
                n157 = local write "retry次數"(w339) -> ()
                n158 = local write "Retry"(w335) -> ()
                n159 = call "Tool RS232 test.vi"("Cmd In"=w340, "VISA resource name"=w305) -> ("error out"=w336:errorcluster, "receive string"=→"Program receive 2":string)  [unwired: 8 in]
                n160 = Unbundle By Name(w336) -> ("status"=w306:bool)
                n161 = Increment(x=w314) -> (x+1=w337:i32)
                n162 = Select(t=w337, s=w306, f=w314) -> (s? t:f=w332:i32)
                n163 = call "Auto Inspection_Status.vi"("Action"=enum16{"Initial", "Write", "Read"}."Write", "DataIn"="PROGRAM", "Station"=Auto_Inspection_Station_Name2."S2Measure", "Data"=Auto_Inspection_Data_Name."CurrentAction") -> ()  [unwired: 9 in, 3 out]
                n164 = Not(x=w306) -> (.not. x?=w307:bool)
                n165 = Greater Or Equal?(x=w332, y=w335) -> (x >= y?=w334:bool)
                n166 = Increment(x=w312) -> (x+1=w333:i32)
                n167 = case shown="False" w334 {
                  tunnel: [errorcluster {"status"=FALSE, "code"=0, "source"=""} ("error constant") errorcluster {"status"=TRUE, "code"=11500, "source"=""} ("error constant")] -> w328
                  tunnel: w332 -> [w349 _]
                  tunnel: [w349 0] -> w310
                  frame False {
                  }
                  frame True {
                  }
                }
                n168 = Select(t=w333, s=w307, f=w312) -> (s? t:f=w311:i32)
                n169 = disable-structure shown="Disabled" {
                  disable-tunnel: [w342 _] -> w327
                  disable-tunnel: w307 -> [w341 _]
                  frame Disabled {
                    n170 = case shown="True" w341 {
                      tunnel: [w343 w346] -> w342
                      frame False {
                        w345 = T7[] [enum."S3 燒入程式 此站執行_34", enum."S3 燒入程式 NG_36"] items=["S2站PC動作中_20", "電流量測完成產品OK_21", "電流量測完成產品NG_22", "S2站Format 執行_23", "S2 Format OK_24", "S2 Format NG_25", "S2站燒入執行_26", "S2站燒入OK_27", "S2站燒入NG_28", "S2站動作完成_29", "S3 PC動作中_30", "S3 Format 此站執行_31", "S3 Format OK_32", "S3 Format NG_33", "S3 燒入程式 此站執行_34", "S3 燒入程式 OK_35", "S3 燒入程式 NG_36", "S3 備用_37", "S3 備用_38", "S3 動作完成_39", "S4 PC動作中_40", "S4 量測完成 產品正常_41", "S4 量測完成 產品NG_42", "S4 Format 此站執行_43", "S4 Format OK_44", "S4 Format NG_45", "S4 燒入 此站不執行_46", "S4 燒入程式 OK_47", "S4 燒入程式 NG_48", "S4 藍芽Scan OK_49", "S4 藍芽Scan NG_50", "S4 動作完成_51", "給PLC要量電流訊號", "給PLC要量電壓訊號"]
                        n171 = call "Set OutputPLC.vi"("Array"=w345, "Address In"=20) -> ("Error Out"=w343:errorcluster[])  [unwired: 9 in]
                      }
                      frame True {
                        w347 = T7[] [enum."S3 燒入程式 此站執行_34", enum."S3 燒入程式 OK_35"] items=["S2站PC動作中_20", "電流量測完成產品OK_21", "電流量測完成產品NG_22", "S2站Format 執行_23", "S2 Format OK_24", "S2 Format NG_25", "S2站燒入執行_26", "S2站燒入OK_27", "S2站燒入NG_28", "S2站動作完成_29", "S3 PC動作中_30", "S3 Format 此站執行_31", "S3 Format OK_32", "S3 Format NG_33", "S3 燒入程式 此站執行_34", "S3 燒入程式 OK_35", "S3 燒入程式 NG_36", "S3 備用_37", "S3 備用_38", "S3 動作完成_39", "S4 PC動作中_40", "S4 量測完成 產品正常_41", "S4 量測完成 產品NG_42", "S4 Format 此站執行_43", "S4 Format OK_44", "S4 Format NG_45", "S4 燒入 此站不執行_46", "S4 燒入程式 OK_47", "S4 燒入程式 NG_48", "S4 藍芽Scan OK_49", "S4 藍芽Scan NG_50", "S4 動作完成_51", "給PLC要量電流訊號", "給PLC要量電壓訊號"]
                        n172 = call "Set OutputPLC.vi"("Array"=w347, "Address In"=20) -> ("Error Out"=w346:errorcluster[])  [unwired: 9 in]
                      }
                    }
                  }
                  frame Enabled {
                  }
                }
                n173 = Select(t="OK" ("DataIn"), s=w307, f="NG" ("DataIn")) -> (s? t:f=w329:string)
                n174 = global read "Main Glb.vi" "Input Registers0-99"() -> (w331:u16[])
                n175 = call "Red PLC InReg.vi"("length"=10, "index"=10, "Input Registers Arr"=w331) -> ("Rad In Reg"=w330:string)  [unwired: 7 in, 1 out]
                n176 = call "Cub Meaasure FGV.vi"("Action"=Table_Save."Write" ("Enum"), "Save Index"=MeasureDisplayTab."Programe(Tool Programe)", "DataIn"=w329, "SN"=w330) -> ()  [unwired: 8 in, 8 out]
                n177 = Merge Errors(w327, w328) -> (w309:errorcluster)
              }
              frame "S1" {
                # "收尋S2站條碼"
                n178 = Index Array(array=w376, index=StationCmdSelect."Command") -> (element=w389:string)
                n179 = call "Retry Num.vi"("String"=w379) -> ("Numeric"=w384:i32, "retry次數"=w388:string[])  [unwired: 9 in]
                n180 = disable-structure shown="Enabled" {
                  disable-tunnel: w355 -> [w404 _]
                  disable-tunnel: [w403 FALSE] -> w353
                  frame Enabled {
                    n181 = call "ToolScanTest.vi"("error in (no error)"=w404, "VISA resource name"=refnum<visa-resource-name> "COM10") -> ("error out"=w400:errorcluster, "read string 6"=w396:string, "Array"=w397:string[])  [unwired: 4 in, 3 out]
                    "Blue Scan receive" <- w396
                    "Array" <- w397
                    n182 = String Length(string=w396) -> (length=w395:i32)
                    n183 = call <vilib>:"Clear Errors.vi"("error in (no error)"=w400) -> ()  [unwired: 5 in, 2 out]
                    n184 = Not Equal?(x=w395, y=0) -> (x != y?=w393:bool)
                    n185 = call "Check Sum Test_01.vi"("Array"=w397) -> ("ToolStringOut_01"=→"S1 ToolStringOut":string, "ChkSum"=→"S1 ChkSum":string, "x = y?"=w399:bool)  [unwired: 8 in]
                    n186 = Not(x=w393) -> (.not. x?=w392:bool)
                    n187 = Not(x=w399) -> (.not. x?=w391:bool)
                    n188 = Or(x=w391, y=w392) -> (x .or. y?=w403:bool)
                  }
                  frame Disabled {
                  }
                }
                n189 = local write "CurrentCmd"(w389) -> ()
                n190 = local write "retry次數"(w388) -> ()
                n191 = local write "Retry"(w384) -> ()
                n192 = call "Tool RS232 test.vi"("error in (no error)"=w355, "Cmd In"=w389, "VISA resource name"=w354) -> ("error out"=w385:errorcluster, "receive string"=→"S1 receive":string)  [unwired: 7 in]
                n193 = Unbundle By Name(w385) -> ("status"=w373:bool)
                n194 = Increment(x=w374) -> (x+1=w386:i32)
                n195 = call "Auto Inspection_Status.vi"("Action"=enum16{"Initial", "Write", "Read"}."Write", "DataIn"="SCAN1", "Station"=Auto_Inspection_Station_Name2."S2Measure", "Data"=Auto_Inspection_Data_Name."CurrentAction") -> ()  [unwired: 9 in, 3 out]
                n196 = Or(x=w353, y=w373) -> (x .or. y?=w356:bool)
                n197 = Select(t=w386, s=w356, f=w374) -> (s? t:f=w381:i32)
                n198 = Greater Or Equal?(x=w381, y=w384) -> (x >= y?=w383:bool)
                n199 = Not(x=w356) -> (.not. x?=w357:bool)
                n200 = case shown="False" w383 {
                  tunnel: [errorcluster {"status"=FALSE, "code"=0, "source"=""} ("error constant") errorcluster {"status"=TRUE, "code"=11500, "source"=""} ("error constant")] -> w359
                  tunnel: w381 -> [w406 _]
                  tunnel: [w406 0] -> w380
                  frame False {
                  }
                  frame True {
                  }
                }
                n201 = Increment(x=w378) -> (x+1=w382:i32)
                n202 = Select(t=w382, s=w357, f=w378) -> (s? t:f=w377:i32)
                n203 = global read "Main Glb.vi" "Input Registers0-99"() -> (w368:u16[])
                n204 = Select(t="OK" ("DataIn"), s=w357, f="NG" ("DataIn")) -> (s? t:f=w360:string)
                n205 = call "Red PLC InReg.vi"("length"=10, "index"=10, "Input Registers Arr"=w368) -> ("Rad In Reg"=w367:string)  [unwired: 7 in, 1 out]
                n206 = call "Cub Meaasure FGV.vi"("Action"=Table_Save."Write" ("Enum"), "Save Index"=MeasureDisplayTab."FSKscanl_315(FSK scan)", "DataIn"=w360, "SN"=w367) -> ()  [unwired: 8 in, 8 out]
                n207 = Merge Errors(w359) -> (w358:errorcluster)
              }
              frame "S2" {
                (unwired) refnum<visa-resource-name> "COM1" ("VISA resource name")
                # "收尋S2站條碼"
                n208 = call "Retry Num.vi"("String"=w435) -> ("Numeric"=w449:i32, "retry次數"=w446:string[])  [unwired: 9 in]
                n209 = Index Array(array=w436, index=StationCmdSelect."Command") -> (element=w429:string)
                n210 = call "ToolScanTest.vi"("error in (no error)"=w437, "VISA resource name"=refnum<visa-resource-name> "COM10") -> ("error out"=w445:errorcluster, "read string 6"=w430:string)  [unwired: 4 in, 4 out]
                "Blue Scan2 receive" <- w430
                n211 = local write "retry次數"(w446) -> ()
                n212 = call "Tool RS232 test.vi"("error in (no error)"=w437, "Cmd In"=w429, "VISA resource name"=w410) -> ("error out"=w452:errorcluster, "receive string"=→"S2 receive":string)  [unwired: 7 in]
                n213 = call <vilib>:"Clear Errors.vi"("error in (no error)"=w445) -> ()  [unwired: 5 in, 2 out]
                n214 = local write "CurrentCmd"(w429) -> ()
                n215 = local write "Retry"(w449) -> ()
                n216 = Unbundle By Name(w452) -> ("status"=w441:bool)
                n217 = String Length(string=w430) -> (length=w444:i32)
                n218 = Not Equal To 0?(x=w444) -> (x != 0?=w443:bool)
                n219 = Not(x=w443) -> (.not. x?=w442:bool)
                n220 = Or(x=w442, y=w441) -> (x .or. y?=w411:bool)
                n221 = Not(x=w411) -> (.not. x?=w412:bool)
                n222 = call "Auto Inspection_Status.vi"("Action"=enum16{"Initial", "Write", "Read"}."Write", "DataIn"="SCAN2", "Station"=Auto_Inspection_Station_Name2."S2Measure", "Data"=Auto_Inspection_Data_Name."CurrentAction") -> ()  [unwired: 9 in, 3 out]
                n223 = Increment(x=w434) -> (x+1=w450:i32)
                n224 = Select(t=w450, s=w411, f=w434) -> (s? t:f=w447:i32)
                n225 = Increment(x=w438) -> (x+1=w451:i32)
                n226 = Greater Or Equal?(x=w447, y=w449) -> (x >= y?=w448:bool)
                n227 = Select(t=w451, s=w412, f=w438) -> (s? t:f=w431:i32)
                n228 = case shown="True" w448 {
                  tunnel: [errorcluster {"status"=FALSE, "code"=0, "source"=""} ("error constant") errorcluster {"status"=TRUE, "code"=11505, "source"=""} ("error constant")] -> w414
                  tunnel: w447 -> [w462 _]
                  tunnel: [w462 0] -> w433
                  frame False {
                  }
                  frame True {
                  }
                }
                n229 = disable-structure shown="Disabled" {
                  disable-tunnel: [w455 _] -> w415
                  disable-tunnel: w412 -> [w454 _]
                  frame Disabled {
                    n230 = case shown="False" w454 {
                      tunnel: [w456 w460] -> w455
                      frame False {
                        w458 = T7[] [enum."S4 量測完成 產品NG_42"] items=["S2站PC動作中_20", "電流量測完成產品OK_21", "電流量測完成產品NG_22", "S2站Format 執行_23", "S2 Format OK_24", "S2 Format NG_25", "S2站燒入執行_26", "S2站燒入OK_27", "S2站燒入NG_28", "S2站動作完成_29", "S3 PC動作中_30", "S3 Format 此站執行_31", "S3 Format OK_32", "S3 Format NG_33", "S3 燒入程式 此站執行_34", "S3 燒入程式 OK_35", "S3 燒入程式 NG_36", "S3 備用_37", "S3 備用_38", "S3 動作完成_39", "S4 PC動作中_40", "S4 量測完成 產品正常_41", "S4 量測完成 產品NG_42", "S4 Format 此站執行_43", "S4 Format OK_44", "S4 Format NG_45", "S4 燒入 此站不執行_46", "S4 燒入程式 OK_47", "S4 燒入程式 NG_48", "S4 藍芽Scan OK_49", "S4 藍芽Scan NG_50", "S4 動作完成_51", "給PLC要量電流訊號", "給PLC要量電壓訊號"]
                        n231 = call "Set OutputPLC.vi"("Array"=w458, "Address In"=20) -> ("Error Out"=w456:errorcluster[])  [unwired: 9 in]
                      }
                      frame True {
                        w459 = T7[] [enum."S4 量測完成 產品正常_41"] items=["S2站PC動作中_20", "電流量測完成產品OK_21", "電流量測完成產品NG_22", "S2站Format 執行_23", "S2 Format OK_24", "S2 Format NG_25", "S2站燒入執行_26", "S2站燒入OK_27", "S2站燒入NG_28", "S2站動作完成_29", "S3 PC動作中_30", "S3 Format 此站執行_31", "S3 Format OK_32", "S3 Format NG_33", "S3 燒入程式 此站執行_34", "S3 燒入程式 OK_35", "S3 燒入程式 NG_36", "S3 備用_37", "S3 備用_38", "S3 動作完成_39", "S4 PC動作中_40", "S4 量測完成 產品正常_41", "S4 量測完成 產品NG_42", "S4 Format 此站執行_43", "S4 Format OK_44", "S4 Format NG_45", "S4 燒入 此站不執行_46", "S4 燒入程式 OK_47", "S4 燒入程式 NG_48", "S4 藍芽Scan OK_49", "S4 藍芽Scan NG_50", "S4 動作完成_51", "給PLC要量電流訊號", "給PLC要量電壓訊號"]
                        n232 = call "Set OutputPLC.vi"("Array"=w459, "Address In"=20) -> ("Error Out"=w460:errorcluster[])  [unwired: 9 in]
                      }
                    }
                  }
                  frame Enabled {
                  }
                }
                n233 = Select(t="OK" ("DataIn"), s=w412, f="NG" ("DataIn")) -> (s? t:f=w416:string)
                n234 = global read "Main Glb.vi" "Input Registers0-99"() -> (w424:u16[])
                n235 = call "Red PLC InReg.vi"("length"=10, "index"=10, "Input Registers Arr"=w424) -> ("Rad In Reg"=w423:string)  [unwired: 7 in, 1 out]
                n236 = call "Cub Meaasure FGV.vi"("Action"=Table_Save."Write" ("Enum"), "Save Index"=MeasureDisplayTab."ASKscan_433(ASK scan)", "DataIn"=w416, "SN"=w423) -> ()  [unwired: 8 in, 8 out]
                n237 = Merge Errors(w415, w414) -> (w413:errorcluster)
              }
              frame "D" {
                n238 = Index Array(array=w476, index=w473) -> (element=w475:dbl)
                n239 = Multiply(x=1000, y=w475) -> (x*y=w474:dbl)
                n240 = Wait (ms)(milliseconds to wait=w474) -> ()  [unwired: 1 out]
                n241 = call "Auto Inspection_Status.vi"("Action"=enum16{"Initial", "Write", "Read"}."Write", "DataIn"="Delay Time", "Station"=Auto_Inspection_Station_Name2."S2Measure", "Data"=Auto_Inspection_Data_Name."CurrentAction") -> ()  [unwired: 9 in, 3 out]
                n242 = Increment(x=w471) -> (x+1=w470:i32)
              }
              frame "T1" {
                (unwired) 10 ("index")
                w503 = u16 3 items=["SYSTem:VERSion?", "SYSTem:ERRor?", "*IDN?", "MEAS:CURR:DC?", "MEAS:VOLT?", "SYSTem:ERRor?"] ("Ringfor34450A")
                w502 = u16 5 items=["SYSTem:VERSion?", "SYSTem:ERRor?", "*IDN?", "MEAS:CURR:DC?", "MEAS:VOLT?", "MEAS:VOLT:DC?"] ("RingforIT8511")
                w500 = u16 1 items=["IT8511", "34450A", "WRBuff"] ("ChangeStatus")
                # "收尋S2站條碼"
                # "量電流"
                n243 = call "Retry Num.vi"("String"=w498) -> ("Numeric"=w508:i32, "retry次數"=w507:string[])  [unwired: 9 in]
                n244 = local write "retry次數"(w507) -> ()
                n245 = call "Auto Inspection_Status.vi"("Action"=enum16{"Initial", "Write", "Read"}."Write", "DataIn"="儀器34450A", "Station"=Auto_Inspection_Station_Name2."S2Measure", "Data"=Auto_Inspection_Data_Name."CurrentAction") -> ()  [unwired: 9 in, 3 out]
                n246 = local write "Retry"(w508) -> ()
                n247 = call "MTool34450A.vi"("Ringfor34450A"=w503, "RingforIT8511"=w502, "VISA resource name"=refnum<visa-resource-name> "USB0::0x2A8D::0xB318::MY59430005::INSTR", "ChangeStatus"=w500) -> ("error out"=w504:errorcluster, 1:"μA"=w483:string, 2:"μA"=→"T1 μA":dbl, "read buffer"=→"T1 buffer":string)  [unwired: 4 in]
                n248 = Unbundle By Name(w504) -> ("status"=w478:bool)
                n249 = Increment(x=w499) -> (x+1=w509:i32)
                n250 = Not(x=w478) -> (.not. x?=w479:bool)
                n251 = Select(t=w509, s=w478, f=w499) -> (s? t:f=w506:i32)
                n252 = Greater Or Equal?(x=w506, y=w508) -> (x >= y?=w505:bool)
                n253 = Increment(x=w497) -> (x+1=w510:i32)
                n254 = Select(t=w510, s=w479, f=w497) -> (s? t:f=w496:i32)
                n255 = case shown="False" w505 {
                  tunnel: [errorcluster {"status"=FALSE, "code"=0, "source"=""} ("error constant") w524] -> w481
                  tunnel: w506 -> [w522 _]
                  tunnel: [w522 0] -> w495
                  tunnel: w504 -> [_ w524]
                  frame False {
                  }
                  frame True {
                  }
                }
                n256 = Select(t=w483, s=w479, f="NG" ("DataIn")) -> (s? t:f=w484:string)
                n257 = global read "Main Glb.vi" "Input Registers0-99"() -> (w490:u16[])
                n258 = disable-structure shown="Disabled" {
                  disable-tunnel: [w515 _] -> w482
                  disable-tunnel: w479 -> [w514 _]
                  frame Disabled {
                    n259 = case shown="True" w514 {
                      tunnel: [w516 w519] -> w515
                      frame False {
                        w518 = T7[] [enum."電流量測完成產品NG_22"] items=["S2站PC動作中_20", "電流量測完成產品OK_21", "電流量測完成產品NG_22", "S2站Format 執行_23", "S2 Format OK_24", "S2 Format NG_25", "S2站燒入執行_26", "S2站燒入OK_27", "S2站燒入NG_28", "S2站動作完成_29", "S3 PC動作中_30", "S3 Format 此站執行_31", "S3 Format OK_32", "S3 Format NG_33", "S3 燒入程式 此站執行_34", "S3 燒入程式 OK_35", "S3 燒入程式 NG_36", "S3 備用_37", "S3 備用_38", "S3 動作完成_39", "S4 PC動作中_40", "S4 量測完成 產品正常_41", "S4 量測完成 產品NG_42", "S4 Format 此站執行_43", "S4 Format OK_44", "S4 Format NG_45", "S4 燒入 此站不執行_46", "S4 燒入程式 OK_47", "S4 燒入程式 NG_48", "S4 藍芽Scan OK_49", "S4 藍芽Scan NG_50", "S4 動作完成_51", "給PLC要量電流訊號", "給PLC要量電壓訊號"]
                        n260 = call "Set OutputPLC.vi"("Array"=w518, "Address In"=20) -> ("Error Out"=w516:errorcluster[])  [unwired: 9 in]
                      }
                      frame True {
                        w520 = T7[] [enum."電流量測完成產品OK_21"] items=["S2站PC動作中_20", "電流量測完成產品OK_21", "電流量測完成產品NG_22", "S2站Format 執行_23", "S2 Format OK_24", "S2 Format NG_25", "S2站燒入執行_26", "S2站燒入OK_27", "S2站燒入NG_28", "S2站動作完成_29", "S3 PC動作中_30", "S3 Format 此站執行_31", "S3 Format OK_32", "S3 Format NG_33", "S3 燒入程式 此站執行_34", "S3 燒入程式 OK_35", "S3 燒入程式 NG_36", "S3 備用_37", "S3 備用_38", "S3 動作完成_39", "S4 PC動作中_40", "S4 量測完成 產品正常_41", "S4 量測完成 產品NG_42", "S4 Format 此站執行_43", "S4 Format OK_44", "S4 Format NG_45", "S4 燒入 此站不執行_46", "S4 燒入程式 OK_47", "S4 燒入程式 NG_48", "S4 藍芽Scan OK_49", "S4 藍芽Scan NG_50", "S4 動作完成_51", "給PLC要量電流訊號", "給PLC要量電壓訊號"]
                        n261 = call "Set OutputPLC.vi"("Array"=w520, "Address In"=20) -> ("Error Out"=w519:errorcluster[])  [unwired: 9 in]
                      }
                    }
                  }
                  frame Enabled {
                  }
                }
                n262 = call "Red PLC InReg.vi"("length"=10, "Input Registers Arr"=w490) -> ("Rad In Reg"=w489:string)  [unwired: 8 in, 1 out]
                n263 = call "Cub Meaasure FGV.vi"("Action"=Table_Save."Write" ("Enum"), "Save Index"=MeasureDisplayTab."耗電流 uA(電流表)", "DataIn"=w484, "SN"=w489) -> ()  [unwired: 8 in, 8 out]
                n264 = Merge Errors(w482, w481) -> (w480:errorcluster)
              }
              frame "T2" {
                w554 = u16 3 items=["SYSTem:VERSion?", "SYSTem:ERRor?", "*IDN?", "MEAS:CURR:DC?", "MEAS:VOLT?", "SYSTem:ERRor?"] ("Ringfor34450A")
                w553 = u16 5 items=["SYSTem:VERSion?", "SYSTem:ERRor?", "*IDN?", "MEAS:CURR:DC?", "MEAS:VOLT?", "MEAS:VOLT:DC?"] ("RingforIT8511")
                w551 = u16 0 items=["IT8511", "34450A", "WRBuff"] ("ChangeStatus")
                # "收尋S2站條碼"
                # "量電壓"
                n265 = call "Auto Inspection_Status.vi"("Action"=enum16{"Initial", "Write", "Read"}."Write", "DataIn"="IT8511", "Station"=Auto_Inspection_Station_Name2."S2Measure", "Data"=Auto_Inspection_Data_Name."CurrentAction") -> ()  [unwired: 9 in, 3 out]
                n266 = call "Retry Num.vi"("String"=w545) -> ("Numeric"=w559:i32, "retry次數"=w558:string[])  [unwired: 9 in]
                n267 = local write "retry次數"(w558) -> ()
                n268 = local write "Retry"(w559) -> ()
                n269 = call "MTool34450A.vi"("Ringfor34450A"=w554, "RingforIT8511"=w553, "VISA resource name"=refnum<visa-resource-name> "COM11", "ChangeStatus"=w551) -> ("error out"=w555:errorcluster, "μA"=→"T2 μA":dbl, "read buffer"=w532:string)  [unwired: 4 in, 1 out]
                "T2 buffer" <- w532
                n270 = Unbundle By Name(w555) -> ("status"=w526:bool)
                n271 = Increment(x=w546) -> (x+1=w528:i32)
                n272 = Not(x=w526) -> (.not. x?=w527:bool)
                n273 = Select(t=w528, s=w526, f=w528) -> (s? t:f=w557:i32)
                n274 = Greater Or Equal?(x=w557, y=w559) -> (x >= y?=w556:bool)
                n275 = Increment(x=w547) -> (x+1=w560:i32)
                n276 = Select(t=w532, s=w527, f="NG" ("DataIn")) -> (s? t:f=w533:string)
                n277 = global read "Main Glb.vi" "Input Registers0-99"() -> (w540:u16[])
                n278 = Select(t=w560, s=w527, f=w547) -> (s? t:f=w548:i32)
                n279 = case shown="False" w556 {
                  tunnel: [errorcluster {"status"=FALSE, "code"=0, "source"=""} ("error constant") w572] -> w530
                  tunnel: w557 -> [w570 _]
                  tunnel: [w570 0] -> w550
                  tunnel: w555 -> [_ w572]
                  frame False {
                  }
                  frame True {
                  }
                }
                n280 = disable-structure shown="Disabled" {
                  disable-tunnel: [w563 _] -> w531
                  disable-tunnel: w527 -> [w562 _]
                  frame Disabled {
                    n281 = case shown="True" w562 {
                      tunnel: [w564 w567] -> w563
                      frame False {
                        w566 = T7[] [enum."S4 量測完成 產品NG_42"] items=["S2站PC動作中_20", "電流量測完成產品OK_21", "電流量測完成產品NG_22", "S2站Format 執行_23", "S2 Format OK_24", "S2 Format NG_25", "S2站燒入執行_26", "S2站燒入OK_27", "S2站燒入NG_28", "S2站動作完成_29", "S3 PC動作中_30", "S3 Format 此站執行_31", "S3 Format OK_32", "S3 Format NG_33", "S3 燒入程式 此站執行_34", "S3 燒入程式 OK_35", "S3 燒入程式 NG_36", "S3 備用_37", "S3 備用_38", "S3 動作完成_39", "S4 PC動作中_40", "S4 量測完成 產品正常_41", "S4 量測完成 產品NG_42", "S4 Format 此站執行_43", "S4 Format OK_44", "S4 Format NG_45", "S4 燒入 此站不執行_46", "S4 燒入程式 OK_47", "S4 燒入程式 NG_48", "S4 藍芽Scan OK_49", "S4 藍芽Scan NG_50", "S4 動作完成_51", "給PLC要量電流訊號", "給PLC要量電壓訊號"]
                        n282 = call "Set OutputPLC.vi"("Array"=w566, "Address In"=20) -> ("Error Out"=w564:errorcluster[])  [unwired: 9 in]
                      }
                      frame True {
                        w568 = T7[] [enum."S4 量測完成 產品正常_41"] items=["S2站PC動作中_20", "電流量測完成產品OK_21", "電流量測完成產品NG_22", "S2站Format 執行_23", "S2 Format OK_24", "S2 Format NG_25", "S2站燒入執行_26", "S2站燒入OK_27", "S2站燒入NG_28", "S2站動作完成_29", "S3 PC動作中_30", "S3 Format 此站執行_31", "S3 Format OK_32", "S3 Format NG_33", "S3 燒入程式 此站執行_34", "S3 燒入程式 OK_35", "S3 燒入程式 NG_36", "S3 備用_37", "S3 備用_38", "S3 動作完成_39", "S4 PC動作中_40", "S4 量測完成 產品正常_41", "S4 量測完成 產品NG_42", "S4 Format 此站執行_43", "S4 Format OK_44", "S4 Format NG_45", "S4 燒入 此站不執行_46", "S4 燒入程式 OK_47", "S4 燒入程式 NG_48", "S4 藍芽Scan OK_49", "S4 藍芽Scan NG_50", "S4 動作完成_51", "給PLC要量電流訊號", "給PLC要量電壓訊號"]
                        n283 = call "Set OutputPLC.vi"("Array"=w568, "Address In"=20) -> ("Error Out"=w567:errorcluster[])  [unwired: 9 in]
                      }
                    }
                  }
                  frame Enabled {
                  }
                }
                n284 = call "Red PLC InReg.vi"("length"=10, "index"=10, "Input Registers Arr"=w540) -> ("Rad In Reg"=w539:string)  [unwired: 7 in, 1 out]
                n285 = call "Cub Meaasure FGV.vi"("Action"=Table_Save."Write" ("Enum"), "Save Index"=MeasureDisplayTab."電池負載電壓", "DataIn"=w533, "SN"=w539) -> ()  [unwired: 8 in, 8 out]
                n286 = Merge Errors(w531, w530) -> (w529:errorcluster)
              }
            }
          }
          frame True {
            w574 = TRUE
            "Boolean" <- w574
          }
        }
        n287 = property class="DigNum (strict)"(reference=w68, "Value"=w67) -> ()  [unwired: 1 in, 2 out]
        n288 = Compound Arithmetic op=OR(w65, w72, "stop") -> (w71:bool)
      }
    }
    frame Enabled {
    }
  }
  n289 = disable-structure shown="Enabled" {
    frame Disabled {
    }
    frame Enabled {
    }
  }
  n290 = disable-structure shown="Enabled" {
    frame Disabled {
      n291 = call "Save Table Test.vi"() -> ()  [unwired: 10 in, 2 out]
    }
    frame Enabled {
    }
  }
